vi "Main Controller.vi"() -> ()   [LabVIEW 2016]
doc: "This is the main real-time VI running on the myRIO device. It handles reading the sensors and writing commands to the motors on the sheepdog robot chassis. Values are displayed to the user on the front panel of this VI."
uses:
  <vilib>/Simulation/Scripting/Companion Diagram/SimConfigNode/SimParams.ctl
  <vilib>/Simulation/Scripting/Companion Diagram/SimConfigNode/_simSolvers.ctl
  <vilib>/Simulation/Implementation/Shared/SIMSCR Execution Mode.ctl
  <vilib>/Platform/TimedLoop/XDataNode/timing_clust.ctl
  <vilib>/Platform/TimedLoop/XDataNode/nitl_modes.ctl
  <vilib>/Platform/TimedLoop/XDataNode/wakeup.ctl
  <vilib>/Simulation/Param Hierarchy/Typedefs/SIMPH Param Control Actions.ctl
  <vilib>/Simulation/Scripting/Editor Utilities/SIM subVI tag data.ctl
  <vilib>/Simulation/Scripting/Editor Utilities/SIM subVI execution type.ctl
  <vilib>/Simulation/Implementation/Shared/NILVSim_ParamChanged.vi
  <vilib>/Simulation/Implementation/Shared/NILVSim_FinishedLate.vi
  <vilib>/Simulation/Implementation/Shared/NILVSIM_BeginStep.vi
  <vilib>/Simulation/Implementation/Shared/SIM Is Init or Final Stage.vi
  <vilib>/Simulation/Implementation/Shared/SIM Fire Discrete SubVI.vi
  <vilib>/Simulation/Utility/Implementation/SIM Halt.vi
  <vilib>/Simulation/Nonlinear/Implementation/NILVSim DeadZone.llb/SIM DeadZone (scalar).vi
  <vilib>/Simulation/Nonlinear/Implementation/NILVSim Saturation.llb/SIM Saturation (scalar).vi
  <vilib>/Simulation/Implementation/Shared/NILVSim_Manager.vi
  <vilib>/Utility/error.llb/Clear Errors.vi
  <vilib>/Simulation/Implementation/Shared/NILVSim_FinalizeModel.vi
  <vilib>/Simulation/Implementation/Shared/SIM Fire Discrete SubVI (Core).vi
  <vilib>/FPGAPlugInAG/myRIO-1900/niLvFpga_Open_myRIO-1900.vi
  <vilib>/rvi/interface/common/dynamic/niFpgaDynamicAddResources.vi
  <vilib>/Simulation/Implementation/Shared/SIM Unbundle Sim Info.vi
  <vilib>/Simulation/Implementation/Shared/SIMSH Read Queue.vi
  <vilib>/Simulation/Implementation/Shared/NILVSim_Initialize.vi
  <vilib>/Utility/error.llb/Error Cluster From Error Code.vi
  <vilib>/rvi/errors/niLvFpgaAdjustHostInterfaceError.vi
  <vilib>/Simulation/Utility/Implementation/NILVSim Get Time and IsAcceptedStep.vi
  <vilib>/Simulation/Implementation/Shared/NILVSim_GetModelError.vi
  <vilib>/Simulation/Implementation/Shared/SIM Bundle Sim Info.vi
  <vilib>/FPGAPlugInAG/Dynamic/niLvFpga_Close_Dynamic.vi
  <vilib>/rvi/interface/nirviOpenFPGA/nirviOpenFPGA.xnode
  FPGA Bitfiles/SheepdogRobotPro_FPGATarget_RobotFPGAUtility_97tw+GI730k.lvbitx
  <vilib>/Simulation/Scripting/Companion Diagram/SimConfigNode/SimDog.xnode
  <vilib>/Simulation/Model Libraries/PID/SIM PID (Academic).vi
  <vilib>/Simulation/Model Libraries/PID/SIM PID.vi
  <vilib>/Platform/TimedLoop/XDataNode/XDataNode.xnode
  <vilib>/rvi/interface/nirviReadWriteControl/nirviReadWriteControl.xnode
  <vilib>/Simulation/Implementation/XNodeFramework/SimXNode/SimX.xnode
  <vilib>/rvi/interface/nirviCloseFPGA/nirviCloseFPGA.xnode
  NiFpgaLv.dll
  <vilib>/rvi/interface/Simulation/niFpgaSimulationCallBeginRW.vi
  <vilib>/Platform/TimedLoop/XDataNode/XDNodeRunTimeDep.lvlib
  <vilib>/Simulation/Implementation/Shared/NI_SIM_Implementation.lvlib
panel:
  out "Motor A Speed":dbl
  out "Motor B Speed":dbl
  in  "Reverse Stop":bool
  out "Wheel Position":dbl
  in  "Reverse Speed":dbl
  out "Boolean array 2":bool[](array[boolean])=[TRUE, TRUE, TRUE, TRUE, TRUE, FALSE, FALSE, FALSE, FALSE, FALSE, FALSE, FALSE, FALSE, FALSE, FALSE, FALSE]
  in  "Use Line Sensor Reverse?":bool
  in  "Throttle Map Reverse":dbl[](array[numeric])=[0.1, 0.1, 0.0, 0.0, -0.1, -0.1]
  in  "Start Robot":bool
  in  "Throttle Map Forwards":dbl[](array[numeric])=[0.1, 0.1, 0.0, 0.0, -0.1, -0.1]
  in  "Use Line Sensor Forwards?":bool
  out "Boolean array":bool[](array[boolean])=[TRUE, TRUE, TRUE, TRUE, TRUE, FALSE, FALSE, FALSE, FALSE, FALSE, FALSE, FALSE, FALSE, FALSE, FALSE, FALSE]
  out "Motor A Speed":dbl
  out "Motor B Speed":dbl
  in  "Forward Stop":bool
  out "Wheel Position":dbl
  in  "Forward Speed":dbl
  # "Reverse Controls"
  # "Forward Controls"
  # "Line Sensor"
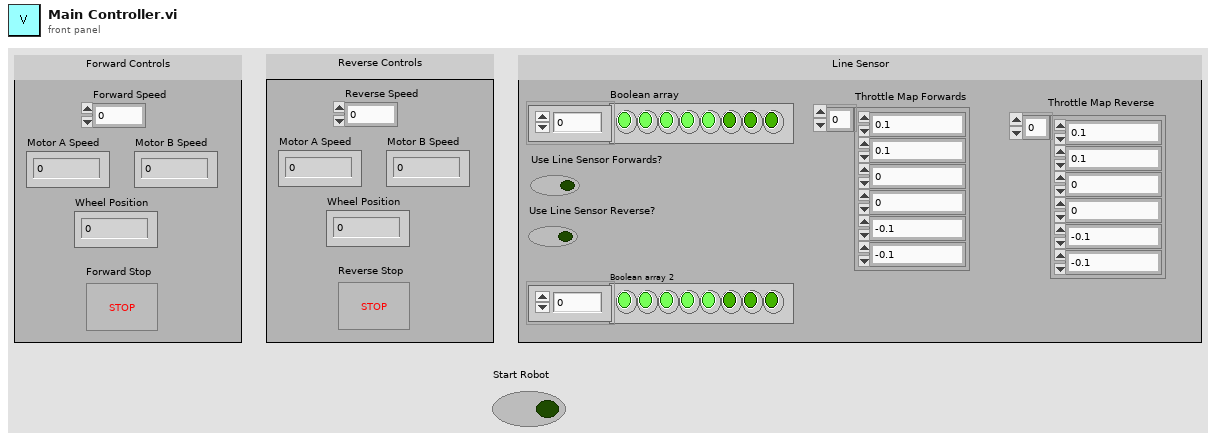
[diagram p1: front panel]
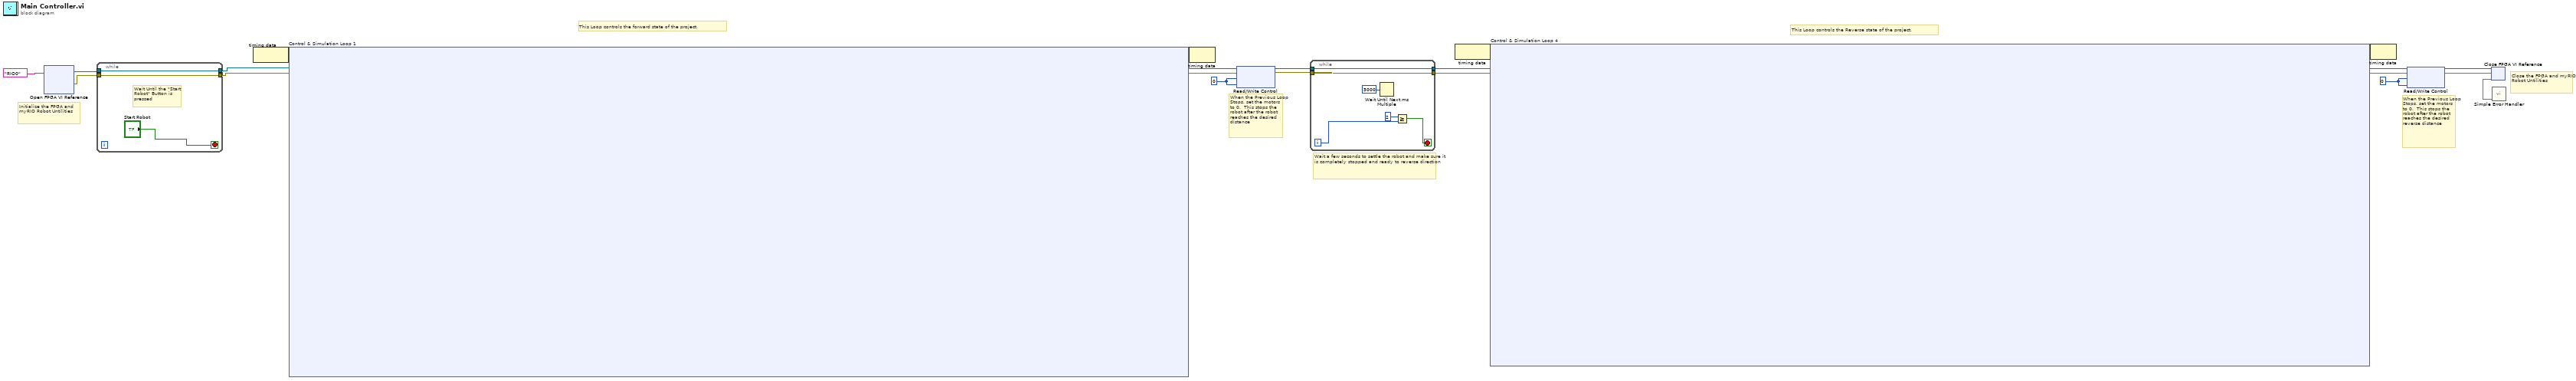
[diagram p0: block diagram]
diagram:
  w11 = 0
  w19 = i16 0 ("Duty Cycle 1")
  # "Close the FPGA and myRIO Robot Untilities"
  # "When the Previous Loop Stops, set the motors to 0.  This stops the robot after the robot reaches the desired  reverse distance"
  # "This Loop controls the Reverse state of the project."
  # "Wait a few seconds to settle the robot and make sure it is completely stopped and ready to reverse direction"
  # "When the Previous Loop Stops, set the motors to 0.  This stops the robot after the robot reaches the desired distance"
  # "This Loop controls the forward state of the project."
  # "Initialize the FPGA and myRIO Robot Untilities"
  n1 = xnode "Open FPGA VI Reference"("resource name"=tag "RIO0") -> ("FPGA VI Reference Out"=w10:refnum<k20>, "error out"=w9:errorcluster)  [unwired: 1 in]
  n2 = while {
    tunnel: w10 -> [w25]
    tunnel: w9 -> [w24]
    tunnel: [w25] -> w8
    tunnel: [w24] -> w7
    stop <- "Start Robot" stop-if-true
    # "Wait Until the \"Start Robot\" Button is pressed"
  }
  n3 = node-c288() -> (w21:variant)  [unwired: 1 in]
  n4 = node-c254 "Control & Simulation Loop 1"(w21, w8, w7) -> (w20:variant, w15:refnum<k20>, w14:errorcluster)
  n5 = node-c288(w20) -> ()  [unwired: 1 out]
  n6 = xnode "Read/Write Control"("FPGA VI Reference In"=w15, "error in"=w14, "Duty Cycle 1"=w11, "Duty Cycle 2"=w11) -> ("FPGA VI Reference Out"=w13:refnum<k20>, "error out"=w12:errorcluster)
  n7 = while {
    tunnel: w13 -> [w27]
    tunnel: w12 -> [w26]
    tunnel: [w27] -> w4
    tunnel: [w26] -> w3
    i -> [w29]
    stop <- w28 stop-if-true
    n8 = Wait Until Next ms Multiple(millisecond multiple=u32 3000) -> ()  [unwired: 1 out]
    n9 = Greater Or Equal?(x=2, y=w29) -> (x >= y?=w28:bool)
  }
  n10 = node-c288() -> (w6:variant)  [unwired: 1 in]
  n11 = node-c254 "Control & Simulation Loop 4"(w6, w4, w3) -> (w5:variant, w1:refnum<k20>, w2:errorcluster)
  n12 = node-c288(w5) -> ()  [unwired: 1 out]
  n13 = xnode "Read/Write Control"("FPGA VI Reference In"=w1, "error in"=w2, "Duty Cycle 1"=w19, "Duty Cycle 2"=w19) -> ("FPGA VI Reference Out"=w18:refnum<k20>, "error out"=w17:errorcluster)
  n14 = xnode "Close FPGA VI Reference"("FPGA VI Reference In"=w18, "error in"=w17) -> ("error out"=w16:errorcluster)
  n15 = call <vilib>:"Simple Error Handler.vi"("error in (no error)"=w16) -> ()  [unwired: 4 in, 5 out]
